vi "Generate Wavforms.vi"(1 "Single Tones.lvclass":refnum<class "Single Tone.lvclass">) -> (0 "Array":waveform(dbl)[](array[waveform]))   [LabVIEW 2017, in "Single Tone.lvclass"]
doc: "This method creates a sine wave output\nbased on the Frequency and Duration values that\nwere acquired by Generate Tone.vi."
uses:
  Single Tone.lvclass
  <vilib>/measure/NI_MABase.lvlib
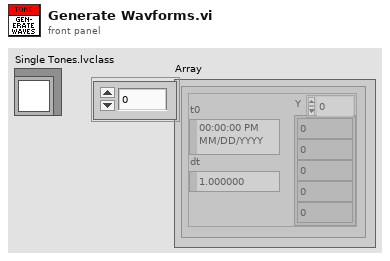
[diagram p1: front panel]
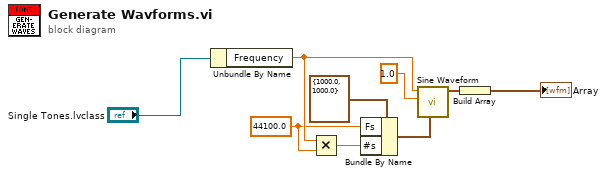
[diagram p0: block diagram]
diagram:
  w3 = 44100.0 ("Fs")
  n1 = Unbundle By Name("Single Tones.lvclass") -> ("Frequency"=w4:dbl)
  n2 = Multiply(x=w4, y=w3) -> (x*y=w5:dbl)
  n3 = Bundle By Name(cluster=cluster{"Fs":dbl, "#s":dbl} {"Fs"=1000.0, "#s"=1000.0} ("sampling info"), "Fs"=w3, "#s"=w5) -> (w6:cluster{"Fs":dbl, "#s":dbl})
  n4 = call <vilib>:"Sine Waveform.vi"("sampling info"=w6, "amplitude"=1.0, "frequency"=w4) -> ("signal out"=w7:waveform(dbl))  [unwired: 7 in, 1 out]
  n5 = Build Array(w7) -> (→"Array":waveform(dbl)[])
